vi "DSF.Engine.Plugin.Rx.Async.vi"(8 "error in (no error)":errorcluster, 11 "Plugin in":refnum<class "DSF.Engine.Plugin.lvclass">) -> (0 "error out":errorcluster, 3 "Plugin out":refnum<class "DSF.Engine.Plugin.lvclass">)   [LabVIEW 2017, in "DSF.Engine.lvlib" / "DSF.Engine.Plugin.lvclass"]
uses:
  DSF.Engine.Plugin.lvclass
  DSF.Engine.Plugin.lvclass/DSF.Engine.Plugin.ctl
  Timing/DSF.Engine.Timing.lvclass/DSF.Engine.Timing.ctl
  Transfer/DSF.Engine.Transfer Group.lvclass/DSF.Engine.Transfer Group.ctl
  Transfer/DSF.Engine.Transfer Group.Get Timing.vi
  Timing/DSF.Engine.Timing.Is Active Cycle.vi
  Transfer/DSF.Engine.Transfer Group.lvclass
  Timing/DSF.Engine.Timing.lvclass
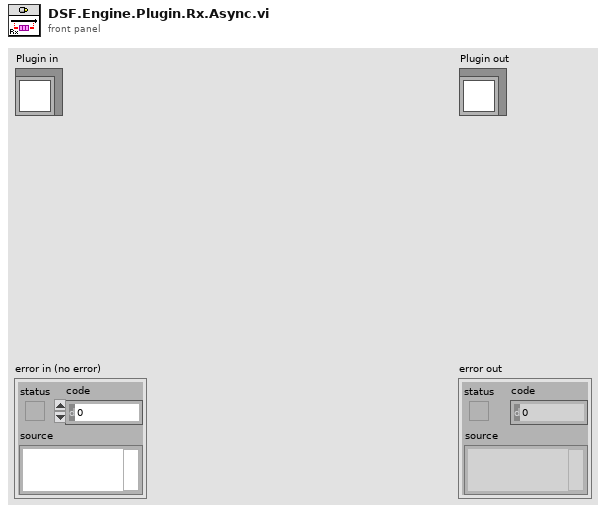
[diagram p1: front panel]
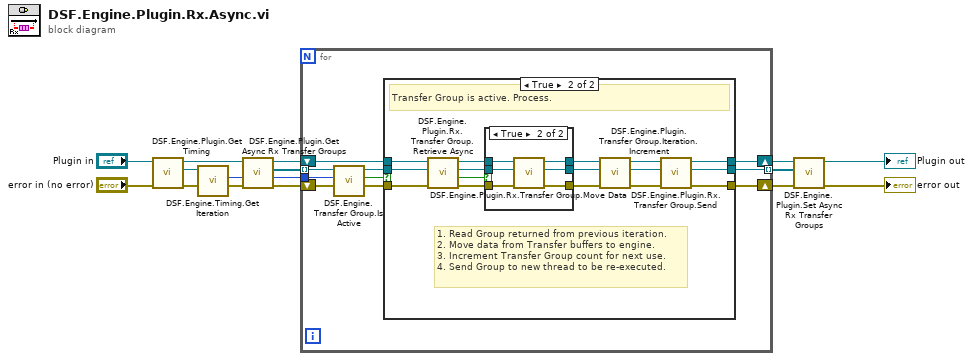
[diagram p0: block diagram]
diagram:
  n1 = call "DSF.Engine.Plugin.Get Timing.vi"("Plugin in"="Plugin in") -> ("Timing"=w5:refnum<class "DSF.Engine.Timing.lvclass">, "Plugin out"=w6:refnum<class "DSF.Engine.Plugin.lvclass">)  [unwired: 9 in]
  n2 = call "DSF.Engine.Timing.Get Iteration.vi"("Timing in"=w5) -> ("Iteration"=w4:u64)  [unwired: 9 in, 1 out]
  n3 = call "DSF.Engine.Plugin.Get Async Rx Transfer Groups.vi"("Plugin in"=w6) -> ("Async Rx Transfer Groups"=w3:refnum<class "DSF.Engine.Transfer Group.lvclass">[], "Plugin out"=w7:refnum<class "DSF.Engine.Plugin.lvclass">)  [unwired: 9 in]
  n4 = for {
    tunnel: w3 -> [w20] mode=indexing
    shift-right: [w13] -> w2
    shift-left: w7 -> [w14]
    tunnel: w4 -> [w19]
    shift-right: [w18] -> w8
    shift-left: "error in (no error)" -> [w17]
    tunnel: [w12] -> w1 mode=indexing
    n5 = call "DSF.Engine.Transfer Group.Is Active.vi"("cycle count"=w19, "Transfer Group in"=w20) -> ("active this cycle?"=w16:bool, "Transfer Group out"=w15:refnum<class "DSF.Engine.Transfer Group.lvclass">)  [unwired: 8 in]
    n6 = case shown="True" w16 {
      tunnel: [w23 w38] -> w18
      tunnel: w17 -> [w23 w36]
      tunnel: w15 -> [w21 w35]
      tunnel: w14 -> [w22 w37]
      tunnel: [w22 w39] -> w13
      tunnel: [w21 w32] -> w12
      frame False {
        # "Transfer Group is not active. Skip."
      }
      frame True {
        # "1. Read Group returned from previous iteration.\n2. Move data from Transfer buffers to engine.\n3. Increment Transfer Group count for next use.\n4. Send Group to new thread to be re-executed."
        # "Transfer Group is active. Process."
        n7 = call "DSF.Engine.Plugin.Rx.Transfer Group.Retrieve Async.vi"("error in (no error)"=w36, "Transfer Group in"=w35, "Plugin in"=w37) -> ("error out"=w25:errorcluster, "move data?"=w26:bool, "Transfer Group out"=w30:refnum<class "DSF.Engine.Transfer Group.lvclass">, "Plugin out"=w31:refnum<class "DSF.Engine.Plugin.lvclass">)  [unwired: 5 in]
        n8 = case shown="True" w26 {
          tunnel: w31 -> [w41 w48]
          tunnel: w30 -> [w42 w47]
          tunnel: [w41 w46] -> w29
          tunnel: [w42 w45] -> w28
          tunnel: [w40 w44] -> w27
          tunnel: w25 -> [w40 w43]
          frame False {
          }
          frame True {
            n9 = call "DSF.Engine.Plugin.Rx.Transfer Group.Move Data.vi"("error in (no error)"=w43, "Transfer Group in"=w47, "Plugin in"=w48) -> ("error out"=w44:errorcluster, "Transfer Group out"=w45:refnum<class "DSF.Engine.Transfer Group.lvclass">, "Plugin out"=w46:refnum<class "DSF.Engine.Plugin.lvclass">)  [unwired: 6 in]
          }
        }
        n10 = call "DSF.Engine.Plugin.Transfer Group.Iteration.Increment.vi"("error in (no error)"=w27, "Transfer Group in"=w28, "Plugin in"=w29) -> ("error out"=w33:errorcluster, "Transfer Group out"=w24:refnum<class "DSF.Engine.Transfer Group.lvclass">, "Plugin out"=w34:refnum<class "DSF.Engine.Plugin.lvclass">)  [unwired: 6 in]
        n11 = call "DSF.Engine.Plugin.Rx.Transfer Group.Send.vi"("error in (no error)"=w33, "Transfer Group in"=w24, "Plugin in"=w34) -> ("error out"=w38:errorcluster, "Transfer Group out"=w32:refnum<class "DSF.Engine.Transfer Group.lvclass">, "Plugin out"=w39:refnum<class "DSF.Engine.Plugin.lvclass">)  [unwired: 6 in]
      }
    }
  }
  "error out" <- w8
  n12 = call "DSF.Engine.Plugin.Set Async Rx Transfer Groups.vi"("Async Rx Transfer Groups"=w1, "Plugin in"=w2) -> ("Plugin out"=→"Plugin out":refnum<class "DSF.Engine.Plugin.lvclass">)  [unwired: 9 in]
